vi "ProcessName.vi"() -> (1 "process name":string="EmsaDataEventCreator")   [LabVIEW 2017, in "EmsaDataEventCreator.lvlib"]
uses:
  <vilib>/addons/InsightCM/Devices/Shared/Emsa/EmsaDataEventCreator/EmsaDataEventCreator.lvlib
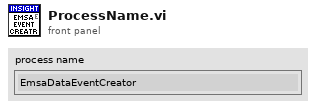
[diagram p1: front panel]
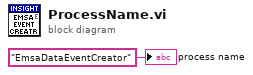
[diagram p0: block diagram]
diagram:
  "process name" <- "EmsaDataEventCreator" ("ProcessName")
